vi "json_parse_constants.vi"(8 "error in (no error)":errorcluster, 11 "data":string) -> (0 "error out":errorcluster, 2 "value":variant, 3 "remaining data":string)   [LabVIEW 2017]
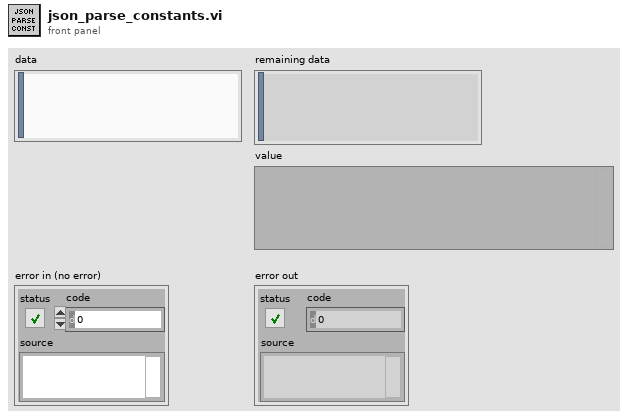
[diagram p1: front panel]
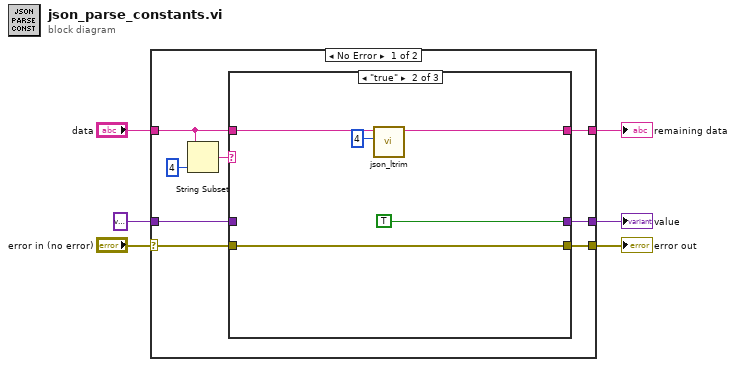
[diagram p0: block diagram]
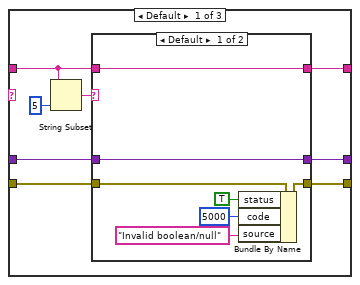
[diagram p2: hidden frame]
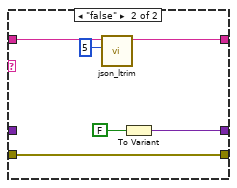
[diagram p3: hidden frame]
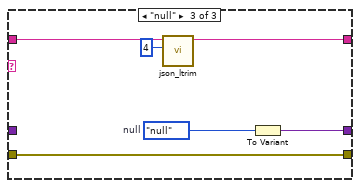
[diagram p4: hidden frame]
diagram:
  n1 = case shown="No Error" "error in (no error)" {
    selector: "error in (no error)" -> [w12 w49]
    tunnel: [w14 w48] -> w6
    tunnel: [w13 w49] -> w5
    tunnel: [w11 w47] -> w3
    tunnel: "data" -> [w10 w48]
    tunnel: variant ("Variant") -> [w7 w47]
    frame No Error {
      n2 = String Subset(string=w10, length (rest)=4 ("length (rest)")) -> (substring=w9:string)  [unwired: 1 in]
      n3 = case shown="\"true\"" w9 {
        tunnel: w10 -> [w16 w37 w42]
        tunnel: [w22 TRUE w45] -> w11
        tunnel: [w21 w36 w41] -> w14
        tunnel: [w19 w39 w46] -> w13
        tunnel: w12 -> [w18 w39 w46]
        tunnel: w7 -> [w20 _ _]
        frame Default {
          n4 = String Subset(string=w16, length (rest)=5 ("length (rest)")) -> (substring=w15:string)  [unwired: 1 in]
          n5 = case shown="Default" w15 {
            tunnel: w16 -> [w29 w31]
            tunnel: [w29 w30] -> w21
            tunnel: [w28 w33] -> w22
            tunnel: w20 -> [w28 _]
            tunnel: [w26 w35] -> w19
            tunnel: w18 -> [w27 w35]
            frame Default {
              n6 = Bundle By Name(cluster=w27, "status"=TRUE, "code"=5000, "source"="Invalid boolean/null") -> (w26:errorcluster)
            }
            frame "false" {
              n7 = call "json_ltrim.vi"("offset (0)"=5 ("length (rest)"), "data"=w31) -> ("left trim whitespace"=w30:string)  [unwired: 9 in]
              n8 = To Variant(anything=FALSE) -> (Variant=w33:variant)
            }
          }
        }
        frame "true" {
          n9 = call "json_ltrim.vi"("offset (0)"=4 ("length (rest)"), "data"=w37) -> ("left trim whitespace"=w36:string)  [unwired: 9 in]
        }
        frame "null" {
          w44 = enum8{"null"}."null"  # null
          n10 = call "json_ltrim.vi"("offset (0)"=4 ("length (rest)"), "data"=w42) -> ("left trim whitespace"=w41:string)  [unwired: 9 in]
          n11 = To Variant(anything=w44) -> (Variant=w45:variant)
        }
      }
    }
    frame Error {
    }
  }
  "remaining data" <- w6
  "error out" <- w5
  "value" <- w3
